vi "CSM - Module Turns Invalid.vi"(3 "CSM Name":string) -> (1 "Turn Invalid (Exit)?":bool)   [LabVIEW 2017, in "Communicable State Machine.lvlib"]
doc: "Checks if a CSM module has already exited. Typically used for a functional loop parallel to the CSM to exit following the CSM loop.\n\nFor modules in CSM Advanced Modes, such as Worker Mode and Chain of Responsibility Mode, the module exit event is triggered only after the last node has exited.\n\n-- <b>Controls</b> --\n\n- <b>CSM Name</b>: CSM module name.\n\n-- <b>Indicators</b> --\n\n- <b>Turn Invalid (Exit)?</b>: Whether the CSM module has already exited."
uses:
  Communicable State Machine.lvlib
  _Support/Typedef/_CSM_List Module Scope.ctl
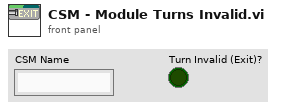
[diagram p1: front panel]
types:
  T1 = typedef "Communicable State Machine.lvlib/_CSM_List Module Scope.ctl" = enum16{"Normal", "System Only", "All"}
  T2 = typedef "Communicable State Machine.lvlib/Priority Queue.ctl" = cluster{"HPriorityQ":refnum<queue>, "LowPriorityQ":refnum<queue>}
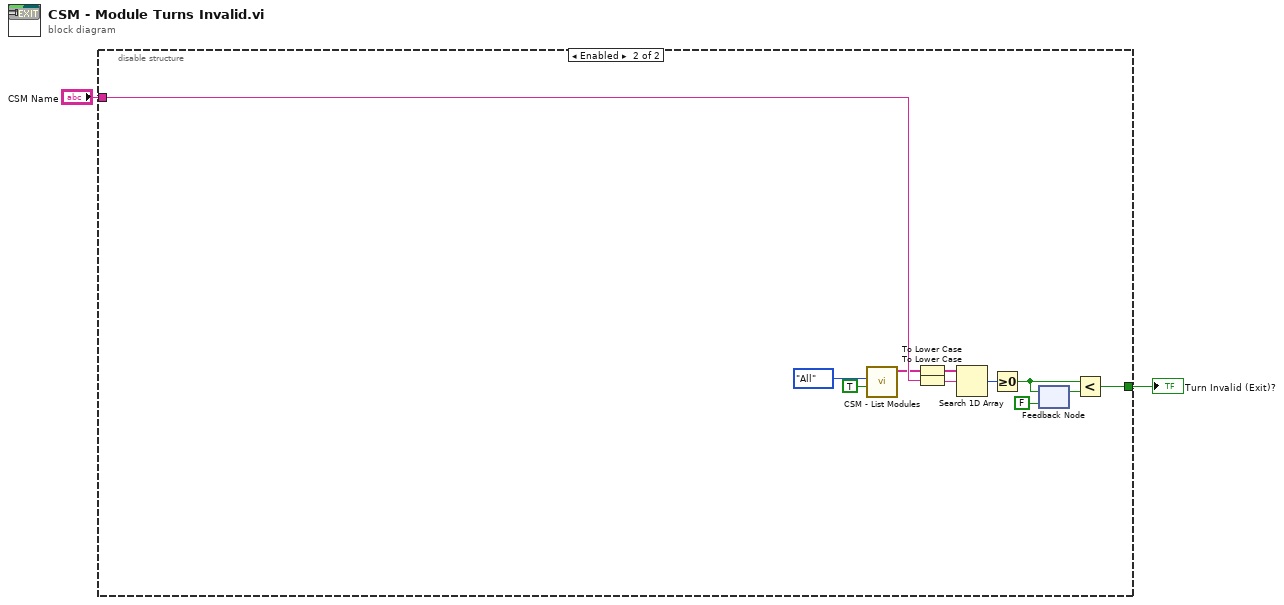
[diagram p0: block diagram]
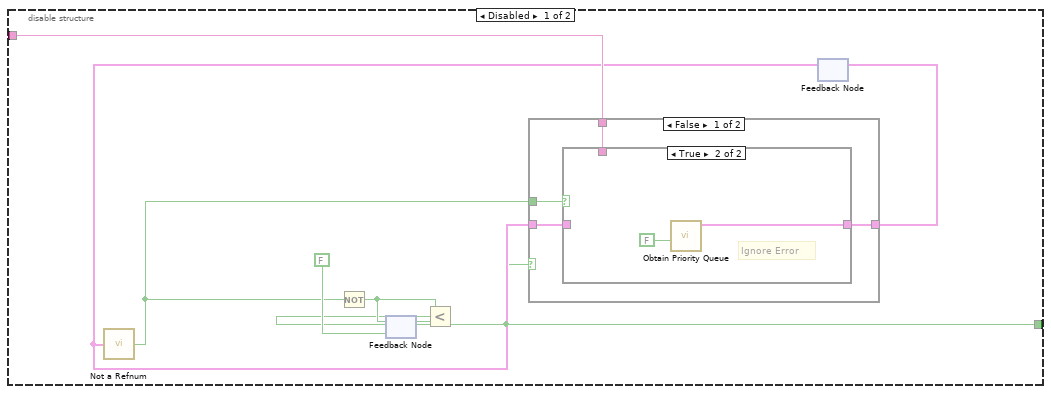
[diagram p2: hidden frame]
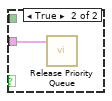
[diagram p4: hidden frame]
diagram:
  n1 = disable-structure shown="Enabled" {
    disable-tunnel: "CSM Name" -> [w10 w29]
    disable-tunnel: [w3 w22] -> w1
    frame Disabled {
      n2 = feedback #1(FALSE) -> (w7:bool)
      n3 = feedback #2() -> (w9:T2)  [unwired: 1 in]
      n4 = call "Not a Refnum.vi"("Priority Queue.lvclass"=w9) -> ("NaN/Path/Refnum?"=w4:bool)  [unwired: 4 in]
      n5 = Not(x=w4) -> (.not. x?=w8:bool)
      n6 = feedback-in #1(w8) -> ()
      n7 = Less?(x=w8, y=w7) -> (x < y?=w3:bool)
      n8 = case shown="False" w3 {
        tunnel: w10 -> [w14 _]
        tunnel: w9 -> [w13 w18]
        tunnel: [w12 _] -> w5
        tunnel: w4 -> [w11 _]
        frame False {
          n9 = case shown="True" w11 {
            tunnel: w14 -> [_ _]
            tunnel: [w15 w16] -> w12
            tunnel: w13 -> [w15 _]
            frame False {
            }
            frame True {
              # "Ignore Error"
              n10 = call "Obtain Priority Queue.vi"("Create If Not Found? (T)"=FALSE ("create if not found? (T)")) -> ("Priority Queue"=w16:T2)  [unwired: 8 in, 2 out]
            }
          }
        }
        frame True {
          n11 = call "Release Priority Queue.vi"("Priority Queue"=w18) -> ()  [unwired: 10 in, 1 out]
        }
      }
      n12 = feedback-in #2(w5) -> ()
    }
    frame Enabled {
      n13 = call "CSM - List Modules.vi"("With Nodes? (F)"=TRUE ("With Instance?"), "Scope (Normal)"=_CSM_List_Module_Scope."All" ("Mode")) -> ("Module Names"=w21:string[])  [unwired: 8 in, 1 out]
      n14 = To Lower Case(string=w21) -> (all lower case string=w28:string[])
      n15 = To Lower Case(string=w29) -> (all lower case string=w27:string)
      n16 = Search 1D Array(1D array=w28, element=w27) -> (index of element=w23:i32)  [unwired: 1 in]
      n17 = Greater Or Equal To 0?(x=w23) -> (x >= 0?=w26:bool)
      n18 = feedback #3(FALSE) -> (w25:bool)
      n19 = feedback-in #3(w26) -> ()
      n20 = Less?(x=w26, y=w25) -> (x < y?=w22:bool)
    }
  }
  "Turn Invalid (Exit)?" <- w1
